vi "Get Bits U8.vi"(9 "Length (1)":u8=1, 10 "Start Index (0)":u8, 11 "Register in":u8 format="%032b") -> (0 "Value":u8 format="%b", 1 "Length out":u8, 2 "Start Index out":u8, 3 "Register out":u8 format="%032b")   [LabVIEW 2016, in "GE 5565PIORC.lvclass"]
uses:
  GE 5565PIORC.lvclass
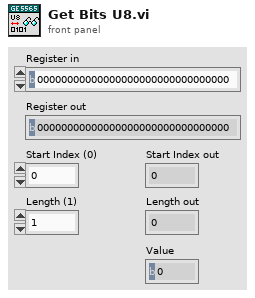
[diagram p1: front panel]
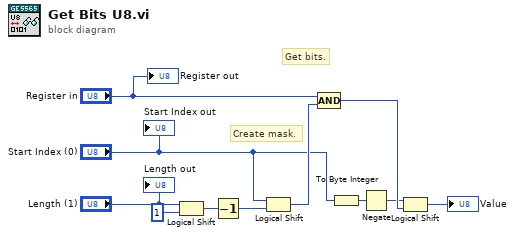
[diagram p0: block diagram]
diagram:
  # "Create mask."
  # "Get bits."
  n1 = Logical Shift(y="Length (1)", x=u8 1) -> (x << y=w8:u8)
  n2 = Decrement(x=w8) -> (x-1=w9:u8)
  n3 = Logical Shift(y="Start Index (0)", x=w9) -> (x << y=w10:u8)
  n4 = Compound Arithmetic op=AND("Register in", w10) -> (w6:u8)
  n5 = To Byte Integer(number="Start Index (0)") -> (8bit integer=w3:i8)
  n6 = Negate(x=w3) -> (-x=w2:i8)
  n7 = Logical Shift(y=w2, x=w6) -> (x << y=→"Value":u8)
  "Register out" <- "Register in"
  "Start Index out" <- "Start Index (0)"
  "Length out" <- "Length (1)"
